vi "2022.12.5-边缘检测-圆.vi"() -> ()   [LabVIEW 2018]
uses:
  <vilib>/vision/Measure.llb/Edge Options.ctl
  <vilib>/vision/Measure.llb/Edge Polarity.ctl
  <vilib>/vision/NI_Vision_Development_Module.lvlib
panel:
  in  "停止":bool
  out "Image":T1(plugin-control)
  out "Coordinate System (duplicate)":T2 {"Measurement System"."Axis Reference" items=["Direct", "Indirect"]; "Measurement System"."Angle (deg)" format="%.2f"; "Measurement System"."Origin"."Y" format="%.2f"; "Measurement System"."Origin"."X" format="%.2f"; "Reference System"."Axis Reference" items=["Direct", "Indirect"]; "Reference System"."Angle (deg)" format="%.2f"; "Reference System"."Origin"."Y" format="%.2f"; "Reference System"."Origin"."X" format="%.2f"}
  out "Fitted Circle":T3 {"Average SNR (dB)" format="%.2f"; "Average Strength" format="%.2f"; "Roundness (Real-World)" format="%.2f"; "Radius (Real-World)" format="%.2f"; "Center (Real-World)"."Y" format="%.2f"; "Center (Real-World)"."X" format="%.2f"; "Radius (Pixels)" format="%.2f"; "Center (Pixels)"."Y" format="%.2f"; "Center (Pixels)"."X" format="%.2f"}
  in  "Options":T6={"Search  Direction"=0, "Edge Options"={"Edge Polarity"=0, "Kernel Size"=3, "Width"=3, "Minimum Edge Strength"=10.0, "Interpolation Type"=enum."Bilinear Fixed", "Data Processing Method"=enum."Average"}, "Show Search Area"=FALSE, "Show Search Lines"=FALSE, "Show Edges Found"=FALSE, "Show Result"=TRUE, "Search Area Color"=65280, "Search Lines Color"=255, "Edge Locations Color"=16776960, "Result Color"=16711680, "Overlay Group Name"=""} {"Search  Direction" items=["Outside to Inside", "Inside to Outside"]; "Edge Options"."Edge Polarity" items=["All Edges", "Rising Edges", "Falling Edges"]; "Edge Options"."Minimum Edge Strength" format="%.2f"; "Edge Options"."Width" step=2; "Edge Options"."Kernel Size" step=2}
  in  "File Path":path
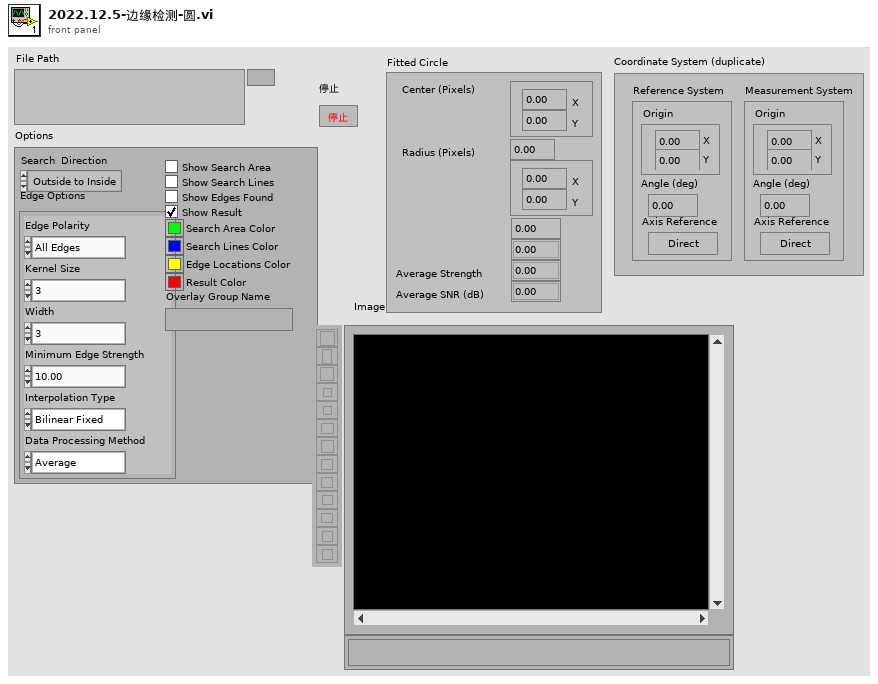
[diagram p1: front panel]
types:
  T1 = typedef "IMAQ Image.ctl" = refnum<image>
  T2 = typedef "IMAQ Coordinate System" = cluster{"Reference System":cluster{"Origin":cluster{"X":sgl, "Y":sgl}, "Angle (deg)":sgl, "Axis Reference":u32}, "Measurement System":cluster{"Origin":cluster{"X":sgl, "Y":sgl}, "Angle (deg)":sgl, "Axis Reference":u32}}
  T3 = cluster{"Center (Pixels)":cluster{"X":sgl, "Y":sgl}, "Radius (Pixels)":dbl, "Center (Real-World)":cluster{"X":sgl, "Y":sgl}, "Radius (Real-World)":dbl, "Roundness (Real-World)":dbl, "Average Strength":dbl, "Average SNR (dB)":dbl}
  T4 = typedef "Edge Options.ctl" = cluster{"Edge Polarity":T5, "Kernel Size":u32, "Width":u32, "Minimum Edge Strength":sgl, "Interpolation Type":enum32{"Zero Order", "Bilinear", "Quadratic", "Cubic", "Bilinear Fixed"}, "Data Processing Method":enum32{"Average", "Median"}}
  T5 = typedef "Edge Polarity.ctl" = u32
  T6 = cluster{"Search  Direction":u32, "Edge Options":T4, "Show Search Area":bool, "Show Search Lines":bool, "Show Edges Found":bool, "Show Result":bool, "Search Area Color":u32, "Search Lines Color":u32, "Edge Locations Color":u32, "Result Color":u32, "Overlay Group Name":string}
  T7 = typedef "Image Type" = u32
  T8 = cluster{"Global Rectangle":i32[], "Contours":cluster{"Contour Type":u32, "ROI Type":u32, "Points":i32[]}[]}
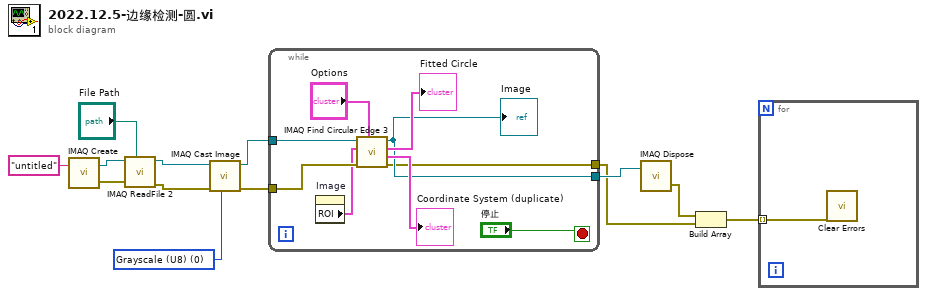
[diagram p0: block diagram]
diagram:
  w7 = T7 0 items=["Grayscale (U8)", "Grayscale (I16)", "Grayscale (SGL)", "Complex (CSG)", "RGB (U32)", "HSL (U32)", "RGB (U64)", "Grayscale (U16)"] ("Image Type")
  n1 = call "IMAQ Create"("Image Name"="untitled") -> ("New Image"=w13:T1, "error out"=w12:errorcluster)  [unwired: 4 in]
  n2 = call "IMAQ ReadFile 2"("File Path"="File Path", "error in (no error)"=w12, "Image"=w13) -> ("error out"=w8:errorcluster, "Image Out"=w9:T1)  [unwired: 4 in, 3 out]
  n3 = call "IMAQ Cast Image"("Image Type"=w7, "error in (no error)"=w8, "Image Src"=w9) -> ("error out"=w5:errorcluster, "Image Dst Out"=w6:T1)  [unwired: 7 in]
  n4 = while {
    tunnel: w6 -> [w22]
    tunnel: w5 -> [w21]
    tunnel: [w17] -> w4
    tunnel: [w14] -> w1
    stop <- "停止" stop-if-true
    n5 = property on="Image" class="ImageControl"() -> ("ROI"=w16:T8)  [unwired: 2 in, 2 out]
    n6 = call "IMAQ Find Circular Edge 3"("Options"="Options", "error in (no error)"=w21, "ROI Descriptor"=w16, "Image"=w22) -> ("error out"=w14:errorcluster, "Coordinate System (duplicate)"=→"Coordinate System (duplicate)":T2, "Fitted Circle"=→"Fitted Circle":T3, "Image Out"=w17:T1)  [unwired: 3 in, 1 out]
    "Image" <- w17
  }
  n7 = call "IMAQ Dispose"("Image"=w4) -> ("error out"=w3:errorcluster)  [unwired: 5 in]
  n8 = Build Array(w3, w1) -> (w2:errorcluster[])
  n9 = for {
    tunnel: w2 -> [w23] mode=indexing
    n10 = call <vilib>:"Clear Errors.vi"("error in (no error)"=w23) -> ()  [unwired: 5 in, 2 out]
  }
